vi "ParStop.vi"(0 "ref in":u64, 11 "error in (no error)":errorcluster) -> (4 "ref out":u64, 6 "return type":i32, 15 "error out":errorcluster)   [LabVIEW 2020, in "Snap7.lvlib"]
uses:
  Snap7.lvlib
  windows/lv_snap7.dll
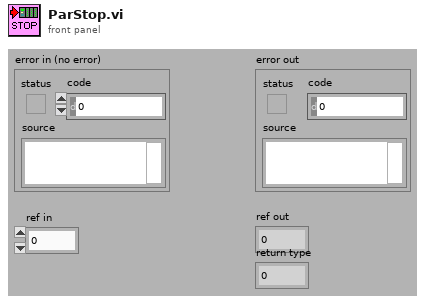
[diagram p1: front panel]
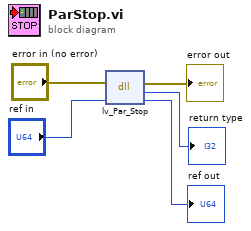
[diagram p0: block diagram]
diagram:
  n1 = dll-call lib="PTH2fabs CUsersFeng项目HLCEPS300-2性能试验台SourcesSnap7libwindowslv_snap7.dll" fn="lv_Par_Stop"(error in="error in (no error)", "Partner"="ref in") -> (error out=→"error out":errorcluster, "return type"=→"return type":i32, "Partner"=→"ref out":u64)  [unwired: 2 in, 1 out]
